vi "Default Directory.vi"(1 "Relative path (.)":path=path "") -> (0 "Default Directory (+ Relative)":path)   [LabVIEW 2012, in "Path Function.lvlib"]
doc: "Returns the default directory + relative path."
uses:
  Path Function.lvlib
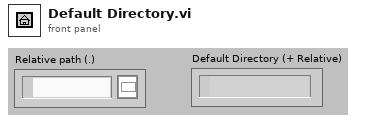
[diagram p1: front panel]
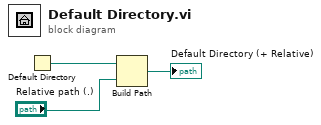
[diagram p0: block diagram]
diagram:
  n1 = Default Directory() -> (w1:path)
  n2 = Build Path(base path=w1, name or relative path="Relative path (.)") -> (appended path=→"Default Directory (+ Relative)":path)
